vi "Run Tx - Mirror Transmit.vi"(7 "Transmit Echo Option":T2, 8 "error in (no error)":errorcluster, 10 "Transmit Value":dbl[](array[numeric]), 11 "Transmit Echo":T1) -> (0 "error out":errorcluster)   [LabVIEW 2016, in "UDP-Custom-Device Engine.lvlib"]
uses:
  UDP-Custom-Device Engine.lvlib
  Shared/Types/Shared - Transmit Echo Options.ctl
  <vilib>/NI/NIVS Inline Async API/_Data Access Engine/Data Access Engine/Types/Write.DVR.ctl
  <vilib>/NI/NIVS Inline Async API/_Data Access Engine/Access Type Classes/Write/Write.lvclass
  <vilib>/NI/NIVS Inline Async API/_Data Access Engine/Access Type Classes/Write/Write.lvclass/Write.ctl
  <vilib>/NI/NIVS Inline Async API/_Data Access Engine/Data Access Engine/Methods/Write.Data.vi
  <vilib>/NI/NIVS Inline Async API/_Data Access Engine/Access Type Classes/Write/Write.ProcessData.vi
  <vilib>/NI/NIVS Inline Async API/_Data Access Engine/Data Access Engine/Data Access Engine.lvclass
  Shared/UDP-Custom-Device Shared.lvlib
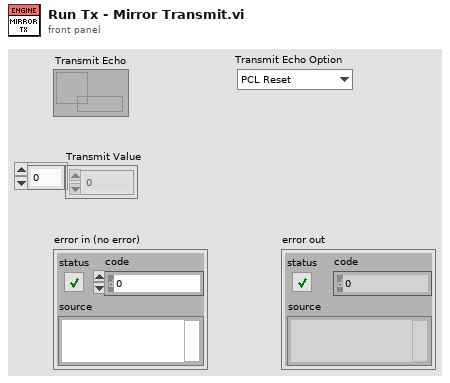
[diagram p1: front panel]
types:
  T1 = typedef "Data Access Engine.lvlib/Data Access Engine.lvclass/Write.DVR.ctl" = refnum<data-value>
  T2 = typedef "UDP-Custom-Device Shared.lvlib/Shared - Transmit Echo Options.ctl" = enum16{"PCL Reset", "Counter", "Mirror"}
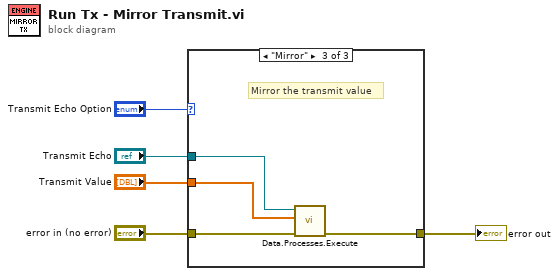
[diagram p0: block diagram]
diagram:
  n1 = case shown="\"Mirror\"" "Transmit Echo Option" {
    tunnel: [w6 w7 w8] -> w5
    tunnel: "error in (no error)" -> [w6 w7 w9]
    tunnel: "Transmit Echo" -> [_ _ w11]
    tunnel: "Transmit Value" -> [_ _ w10]
    frame "PCL Reset", Default {
      # "Do nothing"
    }
    frame "Counter" {
      # "Do nothing"
    }
    frame "Mirror" {
      # "Mirror the transmit value"
      n2 = call-poly <vilib>:"Data.Processes.Execute.vi"("error in (no error)"=w9, "Values"=w10, "Ref"=w11) -> ("error out"=w8:errorcluster)  [unwired: 8 in]
    }
  }
  "error out" <- w5
